vi "UI.vi"(8 "error in (no error)":errorcluster, 11 "View in":refnum<class "View.lvclass">) -> (0 "error out":errorcluster, 3 "View out":refnum<class "View.lvclass">)   [LabVIEW 2020, in "View.lvclass"]
uses:
  View.lvclass
  View.lvclass/View.ctl
panel:
  in  "Integer":i32
  # "Single Page MVC Application\nVIEW"
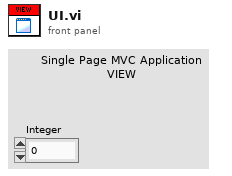
[diagram p1: front panel]
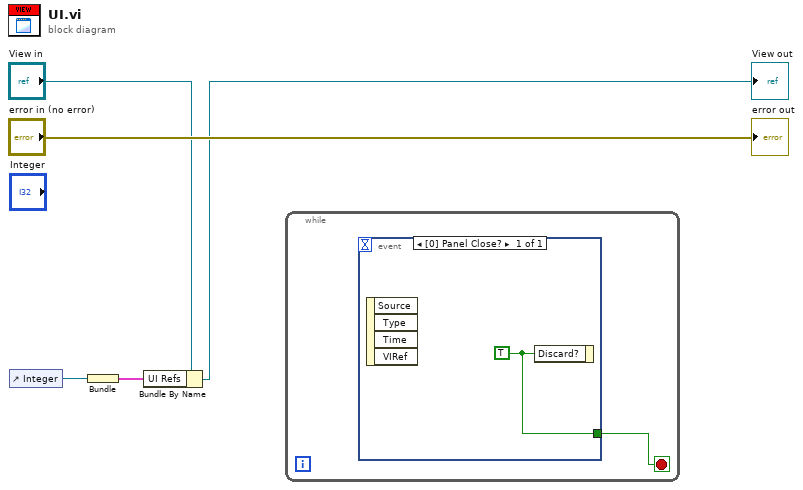
[diagram p0: block diagram]
diagram:
  n1 = control-ref of="Integer"() -> (w4:refnum<vi>)
  n2 = Bundle("Integer"=w4) -> (w2:cluster{"Integer":refnum<vi>})  [unwired: 1 in]
  n3 = Bundle By Name(cluster="View in", "UI Refs"=w2) -> (→"View out":refnum<class "View.lvclass">)
  n4 = while {
    stop <- w6 stop-if-true
    n5 = event shown="[0] Panel Close?" {
      selector: _ -> [_]
      dyn-events: _ -> [_]
      timeout: _ -> [_]
      tunnel: [w7] -> w6
      event Panel Close? {
        w7 = TRUE ("Discard?")
        n6 = event-data() -> ()  [unwired: 1 in, 4 out]
        n7 = event-data("Discard?"=w7) -> ()  [unwired: 1 in, 1 out]
      }
    }
  }
  "error out" <- "error in (no error)"
